vi "dvp Vi Open.vi"(9 "pHandle":u32, 10 "mode":u32(ring) items=["OPEN_OFFLINE", "OPEN_NORMAL"], 11 "index":u32) -> (1 "pHandle out":u32, 3 "function return":u32(ring))   [LabVIEW 2018, in "LabViewDVPCamera.lvlib"]
doc: "LabviewDvp2Api dvpStatus dvpViOpen(dvpUint32 index, dvpOpenMode mode, dvpHandle *pHandle);"
uses:
  LabViewDVPCamera.lvlib
  LabViewDVPCamera/LabViewDVPCamera.dll
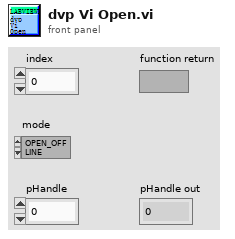
[diagram p1: front panel]
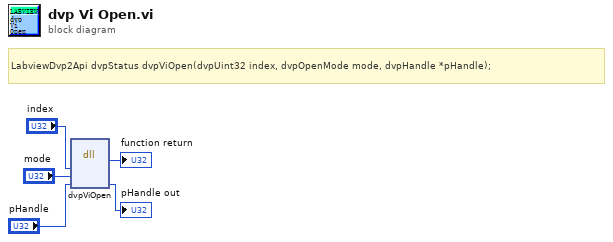
[diagram p0: block diagram]
diagram:
  # "LabviewDvp2Api dvpStatus dvpViOpen(dvpUint32 index, dvpOpenMode mode, dvpHandle *pHandle);"
  n1 = dll-call lib="C:/Program Files (x86)/DVP2 Labview cn 64/Sample/LabViewDVPCamera/LabViewDVPCamera.*" fn="dvpViOpen"("index"="index", "mode"="mode", "pHandle"="pHandle") -> (→"function return":u32, "pHandle"=→"pHandle out":u32)  [unwired: 5 in, 2 out]
